vi "AgilentE363x.vi"(4 "error in":T13, 7 "Command":T14) -> (0 "error out":T13, 3 "Response":T11)   [LabVIEW 2018]
uses:
  MOKO_LabViewLibrary/MokoLowLevel/MokoLowLovelControl/MLLC_Command.ctl
  MOKO_LabViewLibrary/MokoLowLevel/MokoLowLovelControl/MLLC_Error.ctl
  MOKO_LabViewLibrary/MokoLowLevel/MokoLowLovelControl/MLLC_Mode.ctl
  MOKO_LabViewLibrary/MokoLowLevel/MokoLowLovelControl/MLLC_Response.ctl
  MOKO_LabViewLibrary/MokoLowLevel/MokoLowLovelControl/MLLC_DriverName.ctl
  MOKO_LabViewLibrary/MokoLowLevel/MokoLowLovelControl/MLLC_Request.ctl
  MOKO_LabViewLibrary/MokoLowLevel/MokoLowLovelControl/MLLC_ErrorCode.ctl
  MOKO_LabViewLibrary/MokoLowLevel/MokoLowLovelControl/MLLC_ResponseInit.ctl
  MOKO_LabViewLibrary/MokoLowLevel/MokoLowLovelControl/MLLC_ConnectCluster.ctl
  MOKO_LabViewLibrary/MokoLowLevel/MokoLowLovelControl/MLLC_InterfaceType.ctl
  MOKO_LabViewLibrary/MokoLowLevel/MokoLowLovelControl/MLLC_OpenedSession.ctl
  MOKO_LabViewLibrary/MokoLowLevel/MokoLowLovelControl/MLLC_InterfaceSettings.ctl
  MOKO_LabViewLibrary/MokoLowLevel/MokoLowLovelControl/MLLC_InterfaceKind.ctl
panel:
  in  "Settings":T6={"Connect"={"InterfaceType"=enum."VISA", "OpenedSession"="", "InterfaceSettings"={"Interface"=enum."RS232", "EOS 4 read"=enum."LF (\\n)", "EOS 4 write"=enum."LF (\\n)", "TMO, ms"=10000, "Sett"=variant(cluster{"Baud Rate":u32, "Data Bits":u16, "Parity":u16, "Stop Bits":u16, "Flow Control":u16, "Eho":bool} {"Baud Rate"=75, "Data Bits"=0, "Parity"=0, "Stop Bits"=0, "Flow Control"=0, "Eho"=FALSE})}}, "model"="", "VDC Range"=FALSE}
  in  "ResponseInit":T7="E363"
  in  "Error Code":T8=5475
  in  "Request":T9="*IDN?"
  in  "Driver Name":T10="AgilentE363x"
  in  "Mode":T12=enum."Init"
  # "AgilentE363x"
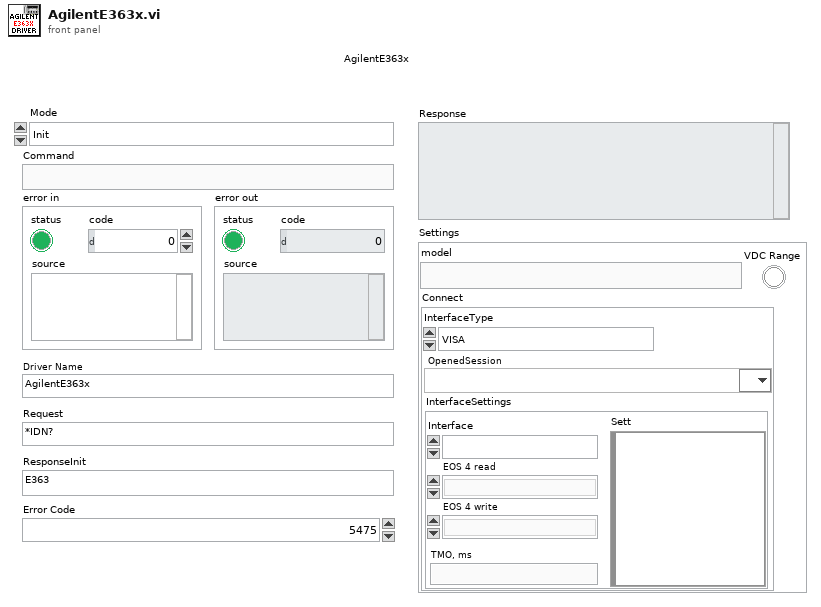
[diagram p1: front panel]
types:
  T1 = typedef "MLLC_ConnectCluster.ctl" = cluster{"InterfaceType":T2, "OpenedSession":T3, "InterfaceSettings":T4}
  T2 = typedef "MLLC_InterfaceType.ctl" = enum16{"VISA", "Prologix USB-GPIB"}
  T3 = typedef "MLLC_OpenedSession.ctl" = refnum<visa-resource-name>
  T4 = typedef "MLLC_InterfaceSettings.ctl" = cluster{"Interface":T5, "EOS 4 read":enum16{"Default (=EOS 4 write)", "CR (\\r)", "LF (\\n)", "None"}, "EOS 4 write":enum16{"CR+LF (\\r\\n)", "CR (\\r)", "LF (\\n)", "None"}, "TMO, ms":i32, "Sett":variant}
  T5 = typedef "MLLC_InterfaceKind.ctl" = enum16{"RS232", "GPIB", "USB", "Ethernet", "another"}
  T6 = cluster{"Connect":T1, "model":string, "VDC Range":bool}
  T7 = typedef "MLLC_ResponseInit.ctl" = string
  T8 = typedef "MLLC_ErrorCode.ctl" = u32
  T9 = typedef "MLLC_Request.ctl" = string
  T10 = typedef "MLLC_DriverName.ctl" = string
  T11 = typedef "MLLC_Response.ctl" = string
  T12 = typedef "MLLC_Mode.ctl" = enum16{"get", "set", "close", "Init", "Check"}
  T13 = typedef "MLLC_Error.ctl" = errorcluster
  T14 = typedef "MLLC_Command.ctl" = string
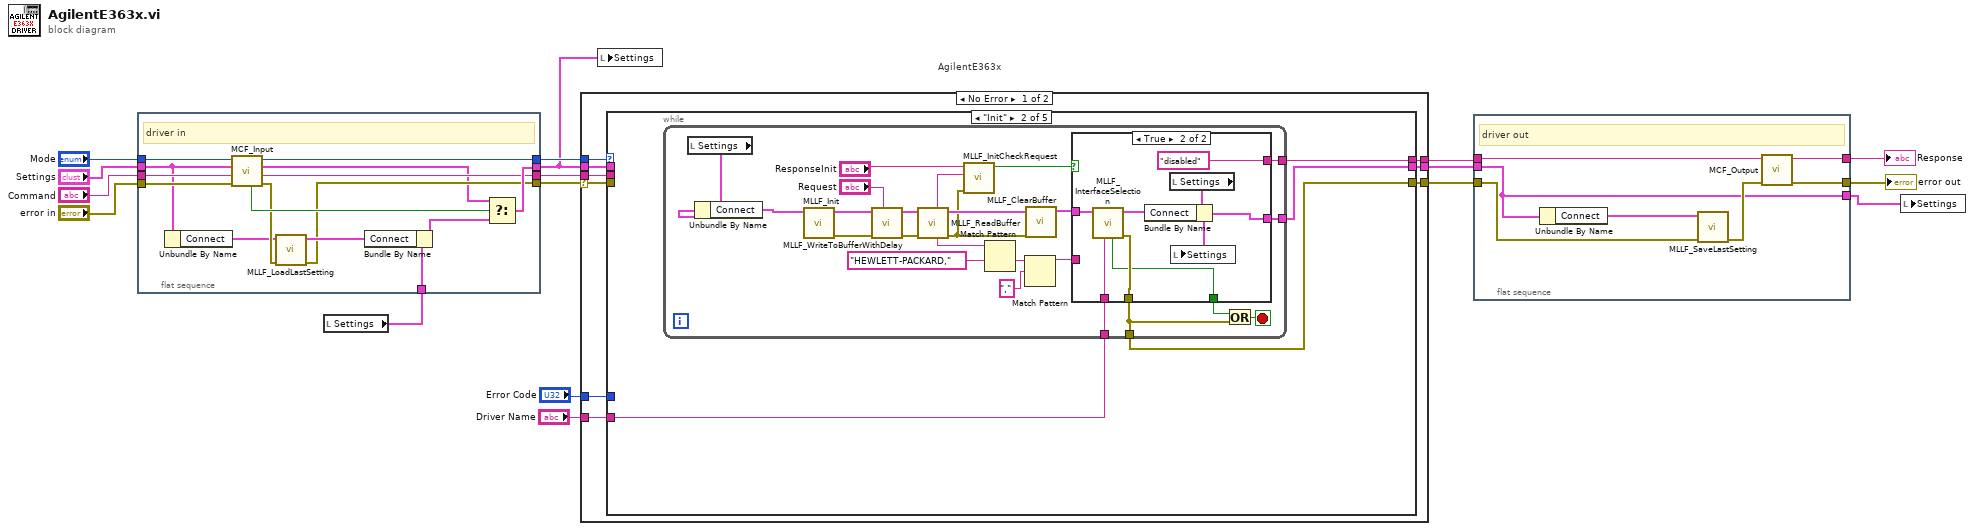
[diagram p0: block diagram]
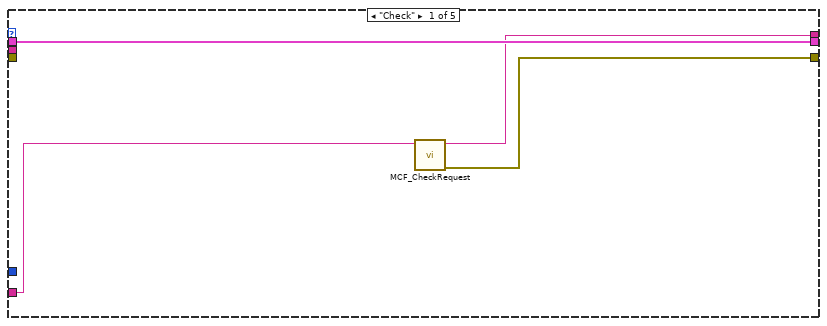
[diagram p2: hidden frame]
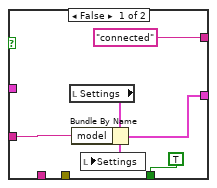
[diagram p3: hidden frame]
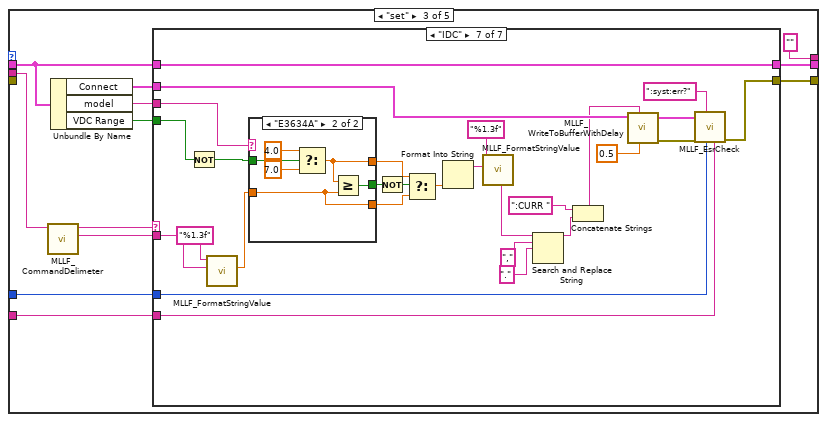
[diagram p4: hidden frame]
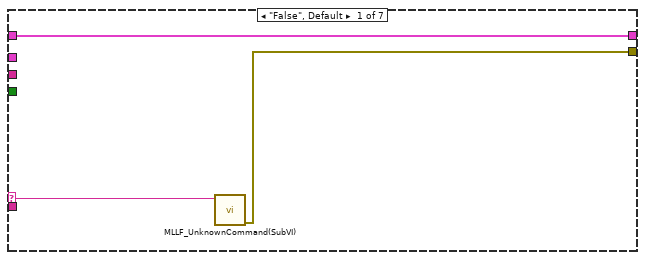
[diagram p5: hidden frame]
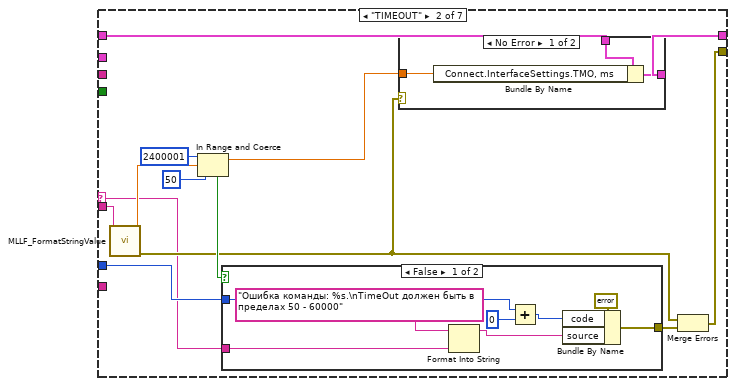
[diagram p6: hidden frame]
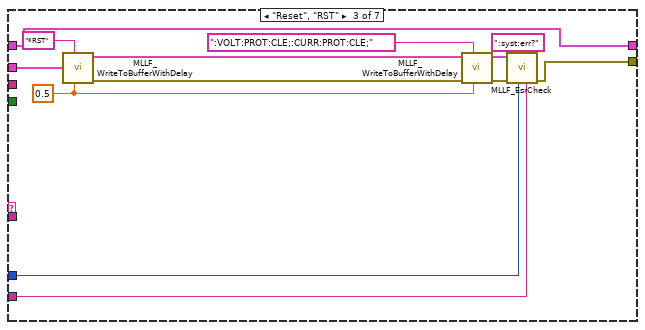
[diagram p9: hidden frame]
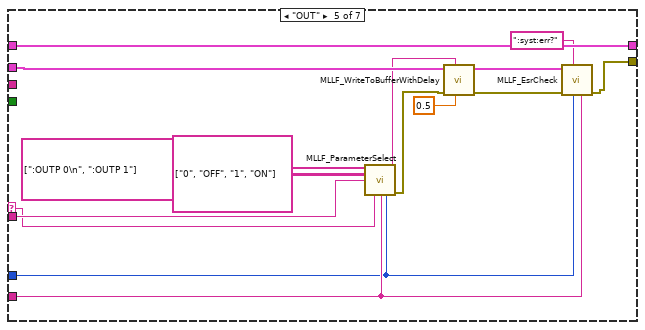
[diagram p11: hidden frame]
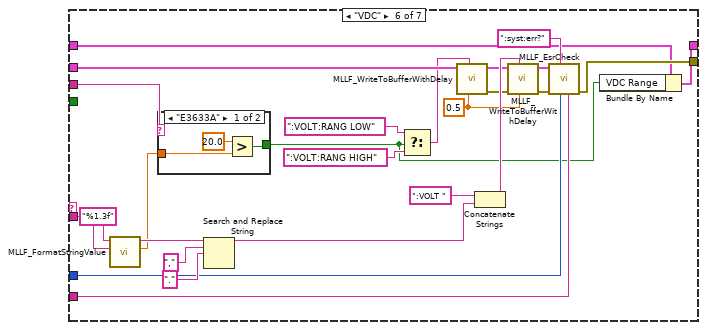
[diagram p12: hidden frame]
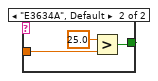
[diagram p13: hidden frame]
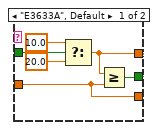
[diagram p14: hidden frame]
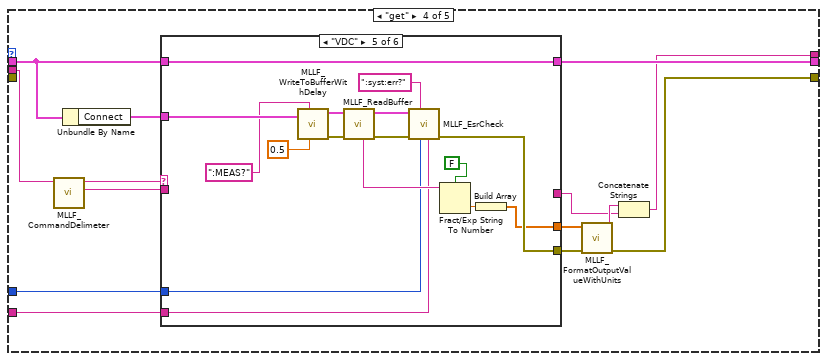
[diagram p15: hidden frame]
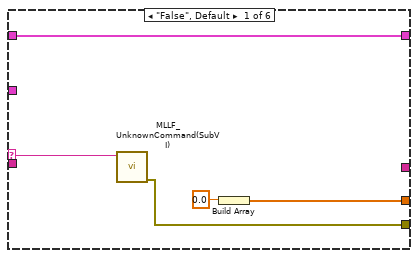
[diagram p16: hidden frame]
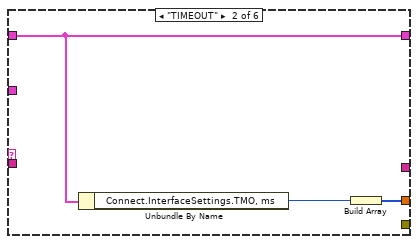
[diagram p17: hidden frame]
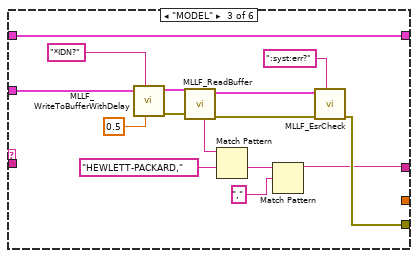
[diagram p18: hidden frame]
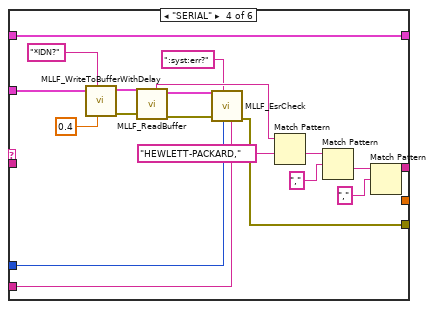
[diagram p19: hidden frame]
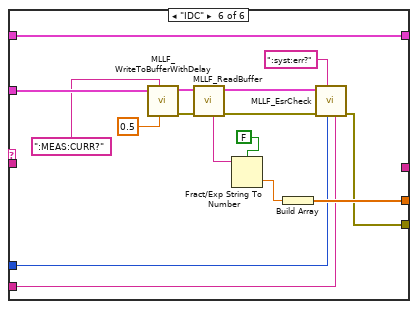
[diagram p20: hidden frame]
diagram:
  # "AgilentE363x"
  n1 = flat-sequence {
    tunnel: [w22] -> w7
    tunnel: [w24] -> w8
    tunnel: "Command" -> [w25]
    tunnel: "Mode" -> [w27]
    tunnel: "Settings" -> [w19]
    tunnel: [w29] -> w2
    tunnel: w3 -> [w28]
    tunnel: "error in" -> [w21]
    tunnel: [w20] -> w9
    frame #0 {
      # "driver in"
      n2 = Unbundle By Name(w19) -> ("Connect"=w18:T1)
      n3 = call "MCF_Input.vi"("Error In"=w21, "Command in"=w25, "Mode in"=w27) -> ("Error Out"=w23:errorcluster, "Command out"=w24:string, "Mode out"=w20:T12, "Boolean"=w26:bool)  [unwired: 5 in]
      n4 = call "MLLF_LoadLastSetting.vi"("Error In"=w23, "DriverConnectCluster in"=w18) -> ("Error Out"=w22:errorcluster, "DriverConnectCluster out"=w30:T1)  [unwired: 8 in]
      n5 = Bundle By Name(cluster=w28, "Connect"=w30) -> (w31:T6)
      n6 = Select(t=w19, s=w26, f=w31) -> (s? t:f=w29:T6)
    }
  }
  n7 = local read "Settings"() -> (w3:T6)
  n8 = case shown="No Error" w7 {
    selector: w7 -> [w36 w319]
    tunnel: [w38 w319] -> w13
    tunnel: w9 -> [w40 _]
    tunnel: [w39 _] -> w15
    tunnel: w8 -> [w37 _]
    tunnel: w2 -> [w33 w318]
    tunnel: "Error Code" -> [w35 _]
    tunnel: "Driver Name" -> [w34 _]
    tunnel: [w32 w318] -> w14
    frame No Error {
      n9 = case shown="\"Init\"" w40 {
        tunnel: [w42 w47 "" ("String") w230 "" ("String")] -> w39
        tunnel: [w43 w45 w85 w226 w316] -> w38
        tunnel: w37 -> [_ _ w88 w229 _]
        tunnel: w36 -> [_ _ _ _ _]
        tunnel: w35 -> [_ _ w96 w237 _]
        tunnel: w34 -> [w41 w48 w93 w236 _]
        tunnel: w33 -> [w44 _ w95 w239 w315]
        tunnel: [w44 w46 w94 w238 w315] -> w32
        frame "Check" {
          n10 = call "MCF_CheckRequest.vi"("Driver Name"=w41) -> ("Error Out"=w43:errorcluster, "Output String"=w42:string)  [unwired: 9 in]
        }
        frame "Init" {
          n11 = while {
            tunnel: [w66] -> w45
            tunnel: w48 -> [w64]
            tunnel: [w54] -> w46
            tunnel: [w53] -> w47
            stop <- w65 stop-if-true
            n12 = local read "Settings"() -> (w71:T6)
            n13 = Unbundle By Name(w71) -> ("Connect"=w68:T1)
            n14 = call "MLLF_Init.vi"("DriverConnect in"=w68) -> ("Error Out"=w62:errorcluster, "DriverConnect out"=w61:T1)  [unwired: 7 in]
            n15 = call "MLLF_WriteToBufferWithDelay.vi"("Command"="Request", "Error In"=w62, "DriverConnect in"=w61) -> ("Error Out"=w70:errorcluster, "DriverConnect out"=w69:T1)  [unwired: 7 in]
            n16 = call "MLLF_ReadBuffer.vi"("Error In"=w70, "DriverConnect in"=w69) -> ("Error Out"=w50:errorcluster, "DriverConnect out"=w60:T1, "String"=w51:string)  [unwired: 6 in]
            n17 = call "MLLF_InitCheckRequest.vi"("error in (no error)"=w50, "Answer"=w51, "Response Init"="ResponseInit") -> ("Design"=w49:bool)  [unwired: 5 in, 3 out]
            n18 = Match Pattern(string=w51, regular expression="HEWLETT-PACKARD," ("search string")) -> (after substring=w57:string)  [unwired: 1 in, 3 out]
            n19 = Match Pattern(string=w57, regular expression="," ("replace string (\"\")")) -> (before substring=w55:string)  [unwired: 1 in, 3 out]
            n20 = call "MLLF_ClearBuffer.vi"("Error In"=w50, "DriverConnect in"=w60) -> ("DriverConnect out"=w59:T1)  [unwired: 6 in, 2 out]
            n21 = case shown="True" w49 {
              tunnel: w59 -> [_ w83]
              tunnel: [TRUE w77] -> w67
              tunnel: [_ w81] -> w66
              tunnel: w64 -> [_ w80]
              tunnel: w55 -> [w74 _]
              tunnel: ["connected" "disabled"] -> w53
              tunnel: [w72 w78] -> w54
              frame False {
                n22 = local read "Settings"() -> (w75:T6)
                n23 = Bundle By Name(cluster=w75, "model"=w74) -> (w72:T6)
                n24 = local write "Settings"(w72) -> ()
              }
              frame True {
                n25 = call "MLLF_InterfaceSelection.vi"("Driver Name"=w80, "DriverConnect in"=w83) -> ("error out"=w81:T13, "DriverConnect out"=w82:T1, "stop init?"=w77:bool)  [unwired: 5 in, 2 out]
                n26 = local read "Settings"() -> (w84:T6)
                n27 = Bundle By Name(cluster=w84, "Connect"=w82) -> (w78:T6)
                n28 = local write "Settings"(w78) -> ()
              }
            }
            n29 = Or(x=w67, y=w66) -> (x .or. y?=w65:bool)
          }
        }
        frame "set" {
          n30 = call "MLLF_CommandDelimeter.vi"("command with param"=w88) -> ("param 1"=w86:string, "command"=w87:string)  [unwired: 6 in, 3 out]
          n31 = Unbundle By Name(w95) -> ("Connect"=w91:T1, "model"=w90:string, "VDC Range"=w89:bool)
          n32 = case shown="\"IDC\"" w87 {
            selector: w87 -> [w98 w100 _ _ w141 _ _]
            tunnel: w86 -> [_ w103 _ _ w149 w178 w210]
            tunnel: [w97 w106 w133 _ w143 w171 w203] -> w85
            tunnel: w96 -> [_ w107 w132 _ w139 w170 w202]
            tunnel: w95 -> [w99 w111 w137 w138 w153 w156 w213]
            tunnel: [w99 w112 w137 w138 w153 w154 w213] -> w94
            tunnel: w91 -> [_ _ w135 _ w152 w164 w212]
            tunnel: w93 -> [_ _ w131 _ w140 w169 w201]
            tunnel: w90 -> [_ _ _ _ _ w157 w197]
            tunnel: w89 -> [_ _ _ _ _ _ w187]
            frame "False", Default {
              n33 = call "MLLF_UnknownCommand(SubVI).vi"("Unknown command"=w98) -> ("error out"=w97:errorcluster)  [unwired: 10 in]
            }
            frame "TIMEOUT" {
              n34 = call "MLLF_FormatStringValue.vi"("String Value"=w103) -> ("error out"=w101:T13, "number"=w102:dbl)  [unwired: 8 in, 1 out]
              n35 = In Range and Coerce(upper limit=2400001, x=w102, lower limit=50) -> (coerced(x)=w108:dbl, In Range?=w104:bool)
              n36 = case shown="False" w104 {
                tunnel: [w119 _] -> w105
                tunnel: w107 -> [w118 _]
                tunnel: w100 -> [w117 _]
                frame False {
                  n37 = Format Into String(format string="Ошибка команды: %s.\nTimeOut должен быть в пределах 50 - 60000", w117) -> (resulting string=w121:string)  [unwired: 2 in, 1 out]
                  n38 = Add(x=w118, y=0) -> (x+y=w122:T8)
                  n39 = Bundle By Name(cluster=errorcluster {"status"=TRUE, "code"=0, "source"=""} ("error out"), "code"=w122, "source"=w121) -> (w119:errorcluster)
                }
                frame True {
                }
              }
              n40 = case shown="No Error" w101 {
                tunnel: [w115 w116] -> w112
                tunnel: w111 -> [w114 w116]
                tunnel: w108 -> [w113 _]
                frame No Error {
                  n41 = Bundle By Name(cluster=w114, "Connect.InterfaceSettings.TMO, ms"=w113) -> (w115:T6)
                }
                frame Error {
                }
              }
              n42 = Merge Errors(w101, w105) -> (w106:errorcluster)
            }
            frame "Reset", "RST" {
              w126 = 0.5 ("Delay Time (s)")
              n43 = call "MLLF_WriteToBufferWithDelay.vi"("Delay Time ( 0,05 s)"=w126, "Command"="*RST" ("write buffer (\"\")"), "DriverConnect in"=w135) -> ("Error Out"=w130:errorcluster, "DriverConnect out"=w129:T1)  [unwired: 7 in]
              n44 = call "MLLF_WriteToBufferWithDelay.vi"("Delay Time ( 0,05 s)"=w126, "Command"=":VOLT:PROT:CLE;:CURR:PROT:CLE;" ("write buffer"), "Error In"=w130, "DriverConnect in"=w129) -> ("Error Out"=w127:errorcluster, "DriverConnect out"=w128:T1)  [unwired: 6 in]
              n45 = call "MLLF_EsrCheck.vi"("Name"=w131, "Error code"=w132, "Error Query"=":syst:err?", "error in"=w127, "DriverConnect in"=w128) -> ("error out"=w133:T13)  [unwired: 5 in, 1 out]
            }
            frame "<----MAIN FUNCTIONS---->" {
            }
            frame "OUT" {
              n46 = call "MLLF_ParameterSelect.vi"("Command to equipment"=string[] [":OUTP 0\n", ":OUTP 1"] ("Names"), "Names"=string[][] [["0", "OFF"], ["1", "ON"]], "Input"=w149, "Command"=w141, "Driver Name"=w140, "Error Code"=w139) -> ("Choice"=w148:string, "Error Out"=w147:errorcluster)  [unwired: 8 in]
              n47 = call "MLLF_WriteToBufferWithDelay.vi"("Delay Time ( 0,05 s)"=0.5 ("Delay Time (s)"), "Command"=w148, "Error In"=w147, "DriverConnect in"=w152) -> ("Error Out"=w142:errorcluster, "DriverConnect out"=w144:T1)  [unwired: 6 in]
              n48 = call "MLLF_EsrCheck.vi"("Name"=w140, "Error code"=w139, "Error Query"=":syst:err?", "error in"=w142, "DriverConnect in"=w144) -> ("error out"=w143:T13)  [unwired: 5 in, 1 out]
            }
            frame "VDC" {
              w158 = 0.5 ("Delay Time (s)")
              n49 = call "MLLF_FormatStringValue.vi"("String Value"=w178, "Format"="%1.3f" ("format string")) -> ("number"=w165:dbl, "String Value Formated"=w175:T14)  [unwired: 7 in, 1 out]
              n50 = case shown="\"E3633A\"" w157 {
                tunnel: w165 -> [w182 w185]
                tunnel: [w180 w183] -> w155
                frame "E3633A" {
                  n51 = Greater?(x=20.0, y=w182) -> (0:w180:bool)
                }
                frame "E3634A", Default {
                  n52 = Greater?(x=25.0, y=w185) -> (0:w183:bool)
                }
              }
              n53 = Search and Replace String(input string=w175, search string=",", replace string="." ("replace string (\"\")")) -> (result string=w167:string)  [unwired: 5 in, 3 out]
              n54 = Select(t=":VOLT:RANG LOW" ("write buffer (\"\")"), s=w155, f=":VOLT:RANG HIGH" ("write buffer (\"\")")) -> (s? t:f=w159:string)
              n55 = call "MLLF_WriteToBufferWithDelay.vi"("Delay Time ( 0,05 s)"=w158, "Command"=w159, "DriverConnect in"=w164) -> ("Error Out"=w162:errorcluster, "DriverConnect out"=w163:T1)  [unwired: 7 in]
              n56 = Concatenate Strings(":VOLT " ("format string"), w167) -> (w166:string)
              n57 = call "MLLF_WriteToBufferWithDelay.vi"("Delay Time ( 0,05 s)"=w158, "Command"=w166, "Error In"=w162, "DriverConnect in"=w163) -> ("Error Out"=w172:errorcluster, "DriverConnect out"=w173:T1)  [unwired: 6 in]
              n58 = call "MLLF_EsrCheck.vi"("Name"=w169, "Error code"=w170, "Error Query"=":syst:err?", "error in"=w172, "DriverConnect in"=w173) -> ("error out"=w171:T13)  [unwired: 5 in, 1 out]
              n59 = Bundle By Name(cluster=w156, "VDC Range"=w155) -> (w154:T6)
            }
            frame "IDC" {
              n60 = Not(x=w187) -> (.not. x?=w186:bool)
              n61 = call "MLLF_FormatStringValue.vi"("String Value"=w210, "Format"="%1.3f" ("format string")) -> ("number"=w196:dbl)  [unwired: 7 in, 2 out]
              n62 = case shown="\"E3634A\"" w197 {
                tunnel: w196 -> [w214 w220]
                tunnel: [w219 w225] -> w194
                tunnel: w186 -> [w218 w224]
                tunnel: [w215 w221] -> w192
                tunnel: [w214 w220] -> w195
                frame "E3633A", Default {
                  n63 = Select(t=10.0, s=w218, f=20.0) -> (s? t:f=w215:dbl)
                  n64 = Greater Or Equal?(x=w215, y=w214) -> (x >= y?=w219:bool)
                }
                frame "E3634A" {
                  n65 = Select(t=4.0, s=w224, f=7.0) -> (s? t:f=w221:dbl)
                  n66 = Greater Or Equal?(x=w221, y=w220) -> (x >= y?=w225:bool)
                }
              }
              n67 = Not(x=w194) -> (.not. x?=w193:bool)
              n68 = Select(t=w192, s=w193, f=w195) -> (s? t:f=w190:dbl)
              n69 = Format Into String(w190) -> (resulting string=w189:string)  [unwired: 3 in, 1 out]
              n70 = call "MLLF_FormatStringValue.vi"("String Value"=w189, "Format"="%1.3f" ("format string")) -> ("String Value Formated"=w188:T14)  [unwired: 7 in, 2 out]
              n71 = Search and Replace String(input string=w188, search string=",", replace string="." ("replace string (\"\")")) -> (result string=w199:string)  [unwired: 5 in, 3 out]
              n72 = Concatenate Strings(":CURR " ("format string"), w199) -> (w198:string)
              n73 = call "MLLF_WriteToBufferWithDelay.vi"("Delay Time ( 0,05 s)"=0.5 ("Delay Time (s)"), "Command"=w198, "DriverConnect in"=w212) -> ("Error Out"=w204:errorcluster, "DriverConnect out"=w205:T1)  [unwired: 7 in]
              n74 = call "MLLF_EsrCheck.vi"("Name"=w201, "Error code"=w202, "Error Query"=":syst:err?", "error in"=w204, "DriverConnect in"=w205) -> ("error out"=w203:T13)  [unwired: 5 in, 1 out]
            }
          }
        }
        frame "get" {
          n75 = call "MLLF_CommandDelimeter.vi"("command with param"=w229) -> ("param 1"=w227:string, "command"=w228:string)  [unwired: 6 in, 3 out]
          n76 = Unbundle By Name(w239) -> ("Connect"=w233:T1)
          n77 = case shown="\"VDC\"" w228 {
            selector: w228 -> [w241 _ _ _ _ _]
            tunnel: w227 -> [_ _ _ _ _ _]
            tunnel: [w240 _ w253 w265 w286 w301] -> w235
            tunnel: w237 -> [_ _ _ w264 w285 w300]
            tunnel: [w244 w247 w262 w281 w297 w313] -> w238
            tunnel: w239 -> [w244 w247 w262 w281 w297 w313]
            tunnel: [w242 w245 _ _ w282 w311] -> w234
            tunnel: w233 -> [_ _ w261 w280 w296 w312]
            tunnel: w236 -> [_ _ _ w263 w284 w299]
            tunnel: [_ _ w248 w270 _ _] -> w231
            frame "False", Default {
              n78 = call "MLLF_UnknownCommand(SubVI).vi"("Unknown command"=w241) -> ("error out"=w240:errorcluster)  [unwired: 10 in]
              n79 = Build Array(0.0 ("TimeOut")) -> (w242:dbl[])
            }
            frame "TIMEOUT" {
              n80 = Unbundle By Name(w247) -> ("Connect.InterfaceSettings.TMO, ms"=w246:i32)
              n81 = Build Array(w246) -> (w245:i32[])
            }
            frame "MODEL" {
              n82 = call "MLLF_WriteToBufferWithDelay.vi"("Delay Time ( 0,05 s)"=0.5 ("Delay Time (s)"), "Command"="*IDN?" ("String"), "DriverConnect in"=w261) -> ("Error Out"=w259:errorcluster, "DriverConnect out"=w260:T1)  [unwired: 7 in]
              n83 = call "MLLF_ReadBuffer.vi"("Error In"=w259, "DriverConnect in"=w260) -> ("Error Out"=w254:errorcluster, "DriverConnect out"=w255:T1, "String"=w252:string)  [unwired: 6 in]
              n84 = Match Pattern(string=w252, regular expression="HEWLETT-PACKARD," ("search string")) -> (after substring=w250:string)  [unwired: 1 in, 3 out]
              n85 = Match Pattern(string=w250, regular expression="," ("replace string (\"\")")) -> (before substring=w248:string)  [unwired: 1 in, 3 out]
              n86 = call "MLLF_EsrCheck.vi"("Error Query"=":syst:err?", "error in"=w254, "DriverConnect in"=w255) -> ("error out"=w253:T13)  [unwired: 7 in, 1 out]
            }
            frame "SERIAL" {
              n87 = call "MLLF_WriteToBufferWithDelay.vi"("Delay Time ( 0,05 s)"=0.4 ("Delay Time (s)"), "Command"="*IDN?" ("String"), "DriverConnect in"=w280) -> ("Error Out"=w278:errorcluster, "DriverConnect out"=w279:T1)  [unwired: 7 in]
              n88 = call "MLLF_ReadBuffer.vi"("Error In"=w278, "DriverConnect in"=w279) -> ("Error Out"=w266:errorcluster, "DriverConnect out"=w267:T1, "String"=w273:string)  [unwired: 6 in]
              n89 = call "MLLF_EsrCheck.vi"("Name"=w263, "Error code"=w264, "Error Query"=":syst:err?", "error in"=w266, "DriverConnect in"=w267) -> ("error out"=w265:T13)  [unwired: 5 in, 1 out]
              n90 = Match Pattern(string=w273, regular expression="HEWLETT-PACKARD," ("search string")) -> (after substring=w274:string)  [unwired: 1 in, 3 out]
              n91 = Match Pattern(string=w274, regular expression="," ("replace string (\"\")")) -> (after substring=w269:string)  [unwired: 1 in, 3 out]
              n92 = Match Pattern(string=w269, regular expression="," ("replace string (\"\")")) -> (before substring=w270:string)  [unwired: 1 in, 3 out]
            }
            frame "VDC" {
              n93 = call "MLLF_WriteToBufferWithDelay.vi"("Delay Time ( 0,05 s)"=0.5 ("Delay Time (s)"), "Command"=":MEAS?" ("format string"), "DriverConnect in"=w296) -> ("Error Out"=w292:errorcluster, "DriverConnect out"=w293:T1)  [unwired: 7 in]
              n94 = call "MLLF_ReadBuffer.vi"("Error In"=w292, "DriverConnect in"=w293) -> ("Error Out"=w287:errorcluster, "DriverConnect out"=w288:T1, "String"=w291:string)  [unwired: 6 in]
              n95 = call "MLLF_EsrCheck.vi"("Name"=w284, "Error code"=w285, "Error Query"=":syst:err?", "error in"=w287, "DriverConnect in"=w288) -> ("error out"=w286:T13)  [unwired: 5 in, 1 out]
              n96 = Fract/Exp String To Number(use system decimal point (T)=FALSE, string=w291) -> (number=w294:dbl)  [unwired: 2 in, 1 out]
              n97 = Build Array(w294) -> (w282:dbl[])
            }
            frame "IDC" {
              n98 = call "MLLF_WriteToBufferWithDelay.vi"("Delay Time ( 0,05 s)"=0.5 ("Delay Time (s)"), "Command"=":MEAS:CURR?" ("format string"), "DriverConnect in"=w312) -> ("Error Out"=w307:errorcluster, "DriverConnect out"=w308:T1)  [unwired: 7 in]
              n99 = call "MLLF_ReadBuffer.vi"("Error In"=w307, "DriverConnect in"=w308) -> ("Error Out"=w302:errorcluster, "DriverConnect out"=w303:T1, "String"=w306:string)  [unwired: 6 in]
              n100 = Fract/Exp String To Number(use system decimal point (T)=FALSE, string=w306) -> (number=w309:dbl)  [unwired: 2 in, 1 out]
              n101 = Build Array(w309) -> (w311:dbl[])
              n102 = call "MLLF_EsrCheck.vi"("Name"=w299, "Error code"=w300, "Error Query"=":syst:err?", "error in"=w302, "DriverConnect in"=w303) -> ("error out"=w301:T13)  [unwired: 5 in, 1 out]
            }
          }
          n103 = call "MLLF_FormatOutputValueWithUnits.vi"("error in"=w235, "ValuesIn"=w234) -> ("error out"=w226:T13, "Result string"=w232:T14)  [unwired: 8 in]
          n104 = Concatenate Strings(w232, w231) -> (w230:string)
        }
        frame "close" {
          n105 = Unbundle By Name(w315) -> ("Connect.OpenedSession"=w317:T3)
          n106 = VISA Close(VISA resource name=w317) -> (error out=w316:errorcluster)  [unwired: 1 in]
        }
      }
    }
    frame Error {
    }
  }
  n107 = local write "Settings"(w2) -> ()
  n108 = flat-sequence {
    tunnel: [w326] -> w12
    tunnel: w15 -> [w325]
    tunnel: w13 -> [w320]
    tunnel: w14 -> [w321]
    tunnel: [w321] -> w10
    tunnel: [w322] -> w11
    frame #0 {
      # "driver out"
      n109 = Unbundle By Name(w321) -> ("Connect"=w324:T1)
      n110 = call "MLLF_SaveLastSetting.vi"("error in"=w320, "DriverConnectCluster in"=w324) -> ("error out"=w323:T13)  [unwired: 8 in, 1 out]
      n111 = call "MCF_Output.vi"("Error In"=w323, "Input"=w325) -> ("Error Out"=w322:errorcluster, "Output"=w326:string)  [unwired: 8 in]
    }
  }
  n112 = local write "Settings"(w10) -> ()
  "error out" <- w11
  "Response" <- w12
